vi "CANBusTestRx.vi"(8 "error in (no error)":errorcluster, 10 "method":string, 11 "Sequence Context In":refnum<k7>) -> (0 "error out":errorcluster, 2 "status":string, 3 "Description":string)   [LabVIEW 2021]
uses:
  <vilib>/addons/TestStand/_TSUtility.llb/TestStand - Get Property Value (String).vi
  <vilib>/NI/JSON Support for LabVIEW/JSON Value/New JSON Value/New JSON (Null).vi
  <vilib>/NI/NI JSONRPC Server Framework/Classes/Client/Format Client Request (Auto-Increment).vi
  <vilib>/NI/NI JSONRPC Server Framework/Classes/Client/JSONRPC Client.lvclass
  <vilib>/NI/JSON Support for LabVIEW/JSON Value/JSON Value.lvclass
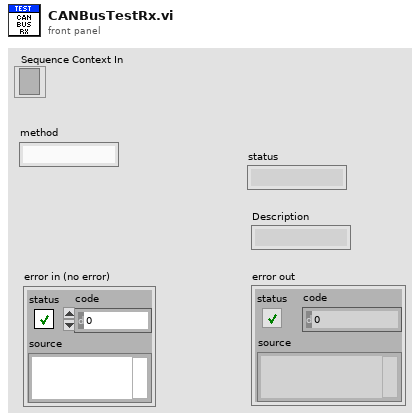
[diagram p1: front panel]
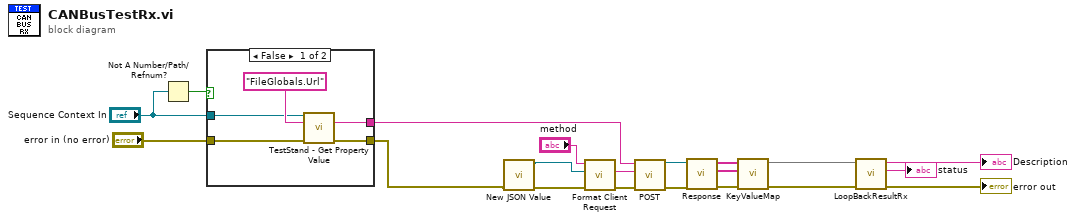
[diagram p0: block diagram]
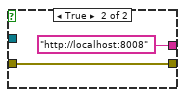
[diagram p2: hidden frame]
diagram:
  n1 = Not A Number/Path/Refnum?(number/path/refnum="Sequence Context In") -> (NaN/Path/Refnum?=w4:bool)
  n2 = case shown="False" w4 {
    tunnel: [w24 "http://localhost:8008" ("Value")] -> w20
    tunnel: [w23 w26] -> w3
    tunnel: "error in (no error)" -> [w22 w26]
    tunnel: "Sequence Context In" -> [w21 _]
    frame False {
      n3 = call-poly <vilib>:"TestStand - Get Property Value.vi"("Sequence Context In"=w21, "Lookup String"="FileGlobals.Url", "error in (no error)"=w22) -> ("Value"=w24:string, "error out"=w23:errorcluster)  [unwired: 10 in, 1 out]
    }
    frame True {
    }
  }
  n4 = call-poly <vilib>:"New JSON Value.vi"("error in (no error)"=w3) -> ("error out"=w2:errorcluster, "JSON Value out"=w1:refnum<class "JSON Value.lvclass">)  [unwired: 9 in]
  n5 = call-poly <vilib>:"Format Client Request.vi"("error in (no error)"=w2, "JSON Value in"=w1, "method"="method") -> ("error out"=w10:errorcluster, "Request String"=w11:string)  [unwired: 7 in]
  n6 = call "POST.vi"("error in (no error)"=w10, "Request String"=w11, "url"=w20) -> ("error out"=w12:errorcluster, "JSON Value out"=w13:refnum<class "JSON Value.lvclass">)  [unwired: 7 in]
  n7 = call "Response.vi"("error in (no error)"=w12, "JSON Value in"=w13) -> ("error out"=w14:errorcluster, "values"=w16:string[], "keys"=w15:string[])  [unwired: 7 in]
  n8 = call "KeyValueMap.vi"("error in"=w14, "values"=w16, "keys"=w15) -> ("error out"=w7:errorcluster, "map out"=w8:map{string, string})  [unwired: 7 in]
  n9 = call "LoopBackResultRx.vi"("error in (no error)"=w7, "map"=w8) -> ("error out"=→"error out":errorcluster, "status"=→"status":string, "description"=→"Description":string)  [unwired: 7 in]
